vi "Read Payload.vi"(8 "error in":errorcluster, 11 "ChanMngOOB_Rx in":refnum<class "ChanMngOOB_Rx.lvclass">) -> (0 "error out":errorcluster, 2 "data":T1 {"Forces"."Force Data" format="%x"; "Connections"."Connection Data" format="%x"}, 3 "ChanMngOOB_Rx out":refnum<class "ChanMngOOB_Rx.lvclass">)   [LabVIEW 2021, in "ChanMngOOB_Rx.lvclass"]
uses:
  ChanMngOOB_Rx.lvclass
  <vilib>/CIF Foundation/CIF Out of Band Commands/CIFOutOfBand.lvclass
  Typedef/Template Payload.ctl
  Typedef/Channel Connection Data.ctl
  Typedef/Channel Fault Data.ctl
  <vilib>/CIF Foundation/CIF Channels Core/ChannelCommon/typedef/New FIFO Instance Configuration.ctl
  <vilib>/CIF Foundation/CIF Channels Core/ChannelCommon/ChannelCommon.lvlib
  Typedef/FIFO Publisher.ctl
  C:/Program Files/National Instruments/LabVIEW 2021/vi.lib/CIF Foundation/CIF Out of Band Commands/CIFOutOfBand.lvclass
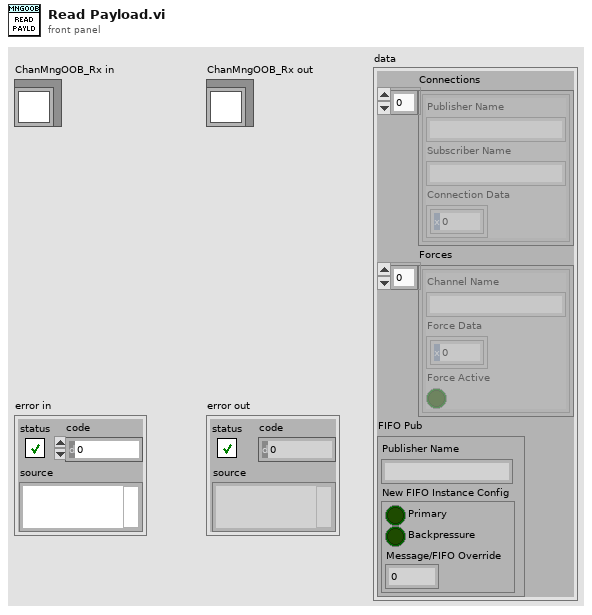
[diagram p1: front panel]
types:
  T1 = typedef "ChanMngOOB_Rx.lvclass/Template Payload.ctl" = cluster{"Connections":T2[], "Forces":T3[], "FIFO Pub":T4}
  T2 = typedef "ChanMngOOB_Rx.lvclass/Channel Connection Data.ctl" = cluster{"Publisher Name":string, "Subscriber Name":string, "Connection Data":u8[]}
  T3 = typedef "ChanMngOOB_Rx.lvclass/Channel Fault Data.ctl" = cluster{"Channel Name":string, "Force Data":u8[], "Force Active":bool}
  T4 = typedef "ChanMngOOB_Rx.lvclass/FIFO Publisher.ctl" = cluster{"Publisher Name":string, "New FIFO Instance Config":T5}
  T5 = typedef "ChannelCommon.lvlib/New FIFO Instance Configuration.ctl" = cluster{"Primary":bool, "Backpressure":bool, "Message/FIFO Override":u32}
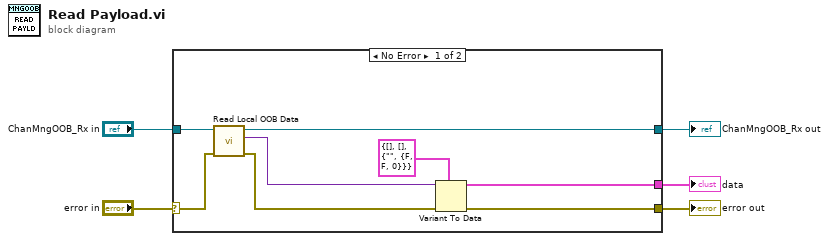
[diagram p0: block diagram]
diagram:
  n1 = case shown="No Error" "error in" {
    selector: "error in" -> [w12 w15]
    tunnel: [w11 w15] -> w5
    tunnel: [w7 w14] -> w4
    tunnel: "ChanMngOOB_Rx in" -> [w13 w14]
    tunnel: [w6 _] -> w1
    frame No Error {
      n2 = call <vilib>:"Read Local OOB Data.vi"("error in"=w12, "OOB in"=w13) -> ("error out"=w10:errorcluster, "Local OOB Data"=w9:variant, "OOB out"=w7:refnum<class "ChanMngOOB_Rx.lvclass">)  [unwired: 7 in]
      n3 = Variant To Data(error in=w10, type=T1 {"Connections"=[], "Forces"=[], "FIFO Pub"={"Publisher Name"="", "New FIFO Instance Config"={"Primary"=FALSE, "Backpressure"=FALSE, "Message/FIFO Override"=0}}}, Variant=w9) -> (data=w6:T1, error out=w11:errorcluster)
    }
    frame Error {
    }
  }
  "error out" <- w5
  "ChanMngOOB_Rx out" <- w4
  "data" <- w1
